vi "CRYAPI Temp Empty.vi"() -> ()   [LabVIEW 2013]
panel:
  in  "NoWait":bool=TRUE
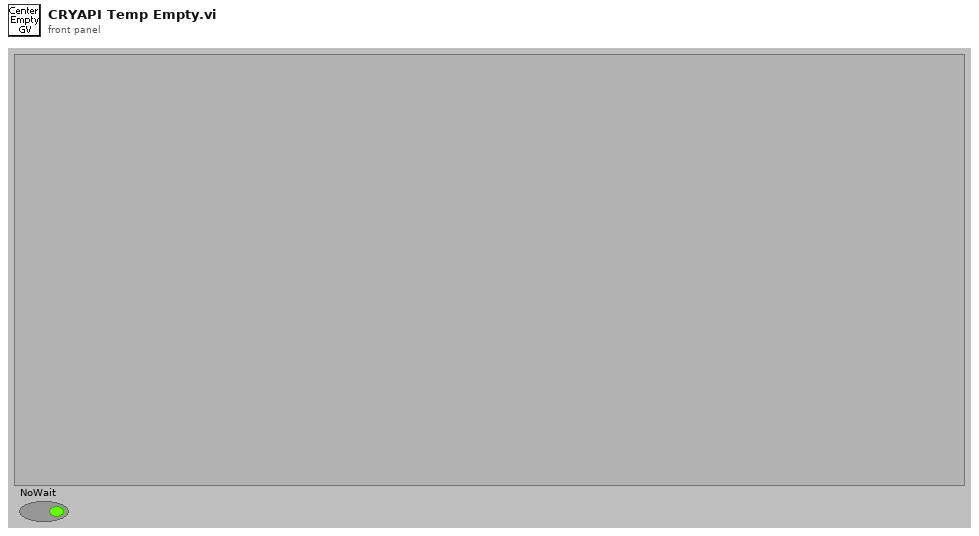
[diagram p1: front panel]
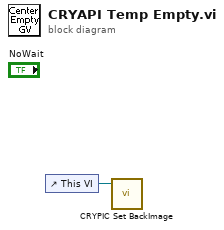
[diagram p0: block diagram]
diagram:
  n1 = control-ref of="This VI"() -> (w1:refnum<vi>)
  n2 = call "CRYPIC Set BackImage.vi"("pVIRef"=w1) -> ()  [unwired: 11 in]
